vi "PH_ImageOperator.allocate or free img space.vi"(0 "i ref in":refnum<vi>, 2 "Allocate?":bool, 5 "error in (no error)":errorcluster) -> (14 "i ref out":refnum<vi>, 19 "error out":errorcluster)   [LabVIEW 2014, in "PH_ImageOperator.lvlib"]
doc: "This VI is forseen to be used in constructor or destructor. If Allocate? = true is chosen, memory space for several images is allocated. If false is chosen, it is freed."
uses:
  PH_ImageOperator.lvlib
  CS_Core/CSSystem/CSSystemLib/CSSystemLib.lvlib
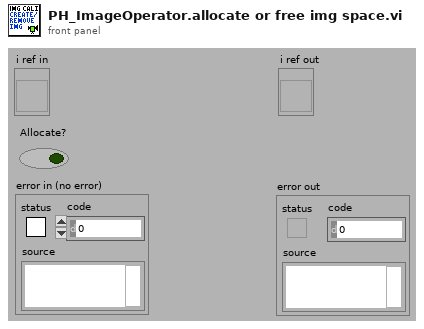
[diagram p1: front panel]
types:
  T1 = typedef "PH_ImageOperator.lvlib/PH_ImageOperator.i attribute.ctl" = cluster{"GUI Refs":cluster{"Delete":refnum<vi>, "Calibration status":refnum<vi>, "BI subtracted":refnum<vi>, "calc Energy":refnum<vi>, "Energy: expected value":refnum<vi>, "Energy: Tolerance":refnum<vi>, "Energy calculated":refnum<vi>, "Energy":refnum<vi>, "calc Beam Anal":refnum<vi>, "Maj Diam 1/esquare":refnum<vi>, "Min Diam 1/esquare":refnum<vi>, "Azi Angle":refnum<vi>, "Min/Maj Diam esquare":refnum<vi>, "Beam analysed":refnum<vi>, "CoG - x":refnum<vi>, "CoG - y":refnum<vi>, "BA: Method":refnum<vi>, "BA: Steps":refnum<vi>, "BA: Factor":refnum<vi>, "calc Traces":refnum<vi>, "Traces: Fit Gauss":refnum<vi>, "Traces calculated":refnum<vi>, "Maj FWHM":refnum<vi>, "Min FWHM":refnum<vi>, "Major Trace":refnum<vi>, "Minor Trace":refnum<vi>, "Maj Fit Order":refnum<vi>, "Min Fit Order":refnum<vi>, "Position calculated":refnum<vi>, "Position":refnum<vi>, "Type":refnum<vi>, "Center":refnum<vi>, "exp - X":refnum<vi>, "exp - Y":refnum<vi>, "Tolerance":refnum<vi>, "f":refnum<vi>, "M":refnum<vi>, "D":refnum<vi>, "q":refnum<vi>, "Dummy Method":refnum<vi>, "Dummy Type":refnum<vi>, "Global On":refnum<vi>, "Traces: No offset":refnum<vi>, "Maj 99%":refnum<vi>, "Min 99%":refnum<vi>, "GUI FF Image":refnum<vi>, "calc Fill Factor":refnum<vi>, "FF calculated":refnum<vi>, "Fill Factor: Filter?":refnum<vi>, "FF: Damage Threshold":refnum<vi>, "FF: Threshold":refnum<vi>, "FF: max allow. Energy":refnum<vi>, "FF: Fillfactor":refnum<vi>, "Calibration data":refnum<vi>}, "List of GUIs":string[], "Calibration":cluster{"Status":T2, "Calibration data":T3, "Calibration Data File":path}, "Final Image":cluster{"BI Subtraction Failure":bool}, "Energy":cluster{"on":bool, "expected value [mJ]":dbl, "Tolerance [%]":dbl, "State":T2, "Energy [mJ]":dbl, "Unit":string, "calculated @":timestamp}, "Beam Analysis":cluster{"on":bool, "Data":T4, "Method":bool, "Steps":i32, "Factor":i32, "ROI":cluster{"Left":i32, "Top":i32, "Right":i32, "Bottom":i32}, "analysed @":timestamp}, "Trace Analysis":cluster{"on":bool, "Fit on":bool, "Maj FWHM":dbl, "Min FWHM":dbl, "Maj Fit Order":i32, "Min Fit Order":i32, "No Offset":bool, "Maj 99%":dbl, "Min 99%":dbl, "Traces":cluster{"XScaleName":string, "Y Scale Minimum":sgl, "Y Scale Maximum":sgl, "X Scale Minimum":sgl, "X Scale Maximum":sgl, "Traces":cluster{"Index":sgl[], "Trace":dbl[]}[]}[], "analysed @":timestamp}, "Position Analysis":cluster{"on":bool, "exp - X":i32, "exp - Y":i32, "focal length [mm]":dbl, "Magnification":dbl, "Delta":dbl, "Theta":dbl, "Tolerance":dbl, "Type":bool, "analysed @":timestamp}, "Fill Factor":cluster{"on":bool, "Filter on?":bool, "Threshold":dbl, "Damage Threshold [J/cm²]":dbl, "Fillfactor":dbl, "Max. allowed Energy [J]":dbl, "calculated @":timestamp}, "Statistician Service ID":i32, "Images":cluster{"Background":T5, "OP":T5, "GUI":T5, "BA: ROI":T5, "Trace: Turn":T5, "FF: Main":T5, "FF: Help":T5, "PSDB: BG":T5, "PSDB: OP":T5, "PSDB: FF":T5}}
  T2 = typedef "PH_StatusHandler.lvlib/PH_StatusHandler.Status.ctl" = i16
  T3 = typedef "PH_ImageCalibrator.lvlib/PH_ImageCalibrator.Calibration Data.ctl" = cluster{"Date":string, "Time":string, "Cam Settings":cluster{"Cam ID":string, "Gain":dbl, "Brightness":dbl, "Shutter":dbl, "Cam Error":bool, "Mode":i32}, "Background Image":cluster{"Image":dbl[][], "Image Error":bool}, "Linear Calibration":cluster{"Calibration Factor":dbl, "not mm or mrad":bool}, "Energy Calibration":cluster{"Calibration Factor":dbl, "no mJ":bool}}
  T4 = typedef "PH_ImageOperator.lvlib/PH_ImageOperator.Beam Analysis Data.ctl" = cluster{"CoG-x":sgl, "CoG-y":sgl, "Maj Dim":dbl, "Min Dim":dbl, "Ellipticity":dbl, "Azimuth Angle [rad]":dbl, "Azi Angle rel to Maj?":bool}
  T5 = typedef "IMAQ Image.ctl" = refnum<image>
  T6 = cluster{"Background":T5, "OP":T5, "GUI":T5, "BA: ROI":T5, "Trace: Turn":T5, "FF: Main":T5, "FF: Help":T5, "PSDB: BG":T5, "PSDB: OP":T5, "PSDB: FF":T5}
  T7 = typedef "Image Type" = u32
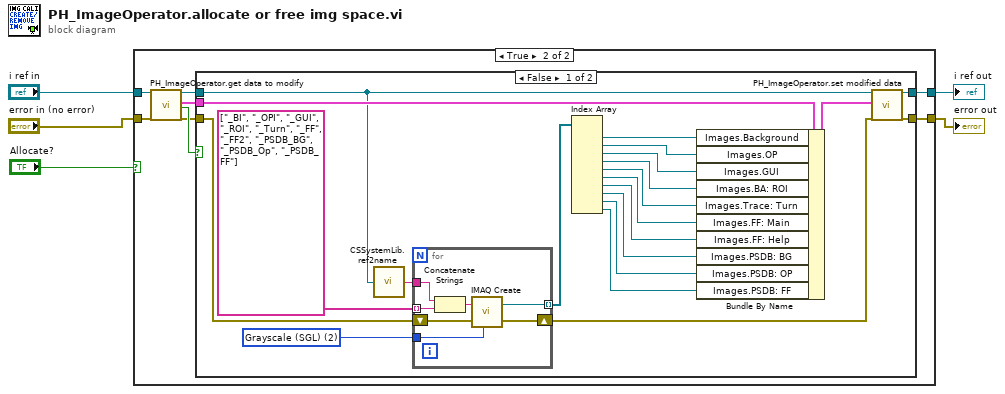
[diagram p0: block diagram]
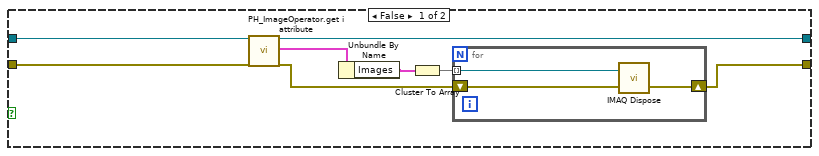
[diagram p2: hidden frame]
diagram:
  n1 = case shown="True" "Allocate?" {
    tunnel: [w8 w23] -> w5
    tunnel: [w10 w22] -> w4
    tunnel: "error in (no error)" -> [w13 w19]
    tunnel: "i ref in" -> [w12 w18]
    frame False {
      n2 = call "PH_ImageOperator.get i attribute.vi"("i ref in"=w12, "error in (no error)"=w13) -> ("i ref out"=w10:refnum<vi>, "i attribute"=w11:T1, "error out"=w9:errorcluster)  [unwired: 15 in]
      n3 = Unbundle By Name(w11) -> ("Images"=w7:T6)
      n4 = Cluster To Array(cluster=w7) -> (array=w6:T5[])
      n5 = for {
        shift-right: [w15] -> w8
        shift-left: w9 -> [w16]
        tunnel: w6 -> [w14] mode=indexing
        n6 = call "IMAQ Dispose"("Image"=w14, "error in (no error)"=w16) -> ("error out"=w15:errorcluster)  [unwired: 4 in]
      }
    }
    frame True {
      n7 = call "PH_ImageOperator.get data to modify.vi"("i ref in"=w18, "error in (no error)"=w19) -> ("i ref out"=w21:refnum<vi>, "i attribute"=w17:T1, "timed out"=w24:bool, "error out"=w20:errorcluster)  [unwired: 14 in]
      n8 = case shown="False" w24 {
        tunnel: w20 -> [w40 w53]
        tunnel: w21 -> [w32 w54]
        tunnel: [w45 w54] -> w22
        tunnel: [w44 w53] -> w23
        tunnel: w17 -> [w43 _]
        frame False {
          w35 = T7 2 items=["Grayscale (U8)", "Grayscale (I16)", "Grayscale (SGL)", "Complex (CSG)", "RGB (U32)", "HSL (U32)", "RGB (U64)"] ("Image Type")
          n9 = call "CSSystemLib.ref2name.vi"("obj refnum"=w32) -> ("name"=w31:string)
          n10 = for {
            shift-right: [w52] -> w41
            shift-left: w40 -> [w51]
            tunnel: [w46] -> w39 mode=indexing
            tunnel: string[] ["_BI", "_OPI", "_GUI", "_ROI", "_Turn", "_FF", "_FF2", "_PSDB_BG", "_PSDB_Op", "_PSDB_FF"] -> [w48] mode=indexing
            tunnel: w35 -> [w50]
            tunnel: w31 -> [w49]
            n11 = Concatenate Strings(w49, w48) -> (w47:string)
            n12 = call "IMAQ Create"("Image Name"=w47, "Image Type"=w50, "error in (no error)"=w51) -> ("New Image"=w46:T5, "error out"=w52:errorcluster)  [unwired: 2 in]
          }
          n13 = Index Array(array=w39) -> (element #1=w37:T5, element #2=w36:T5, element #3=w34:T5, element #4=w33:T5, element #5=w30:T5, element #6=w29:T5, element #7=w28:T5, element #8=w27:T5, element #9=w26:T5, element #10=w25:T5)  [unwired: 10 in]
          n14 = Bundle By Name(cluster=w43, "Images.Background"=w37, "Images.OP"=w36, "Images.GUI"=w34, "Images.BA: ROI"=w33, "Images.Trace: Turn"=w30, "Images.FF: Main"=w29, "Images.FF: Help"=w28, "Images.PSDB: BG"=w27, "Images.PSDB: OP"=w26, "Images.PSDB: FF"=w25) -> (w42:T1)
          n15 = call "PH_ImageOperator.set modified data.vi"("i ref in"=w32, "i attribute"=w42, "error in (no error)"=w41) -> ("i ref out"=w45:refnum<vi>, "error out"=w44:errorcluster)  [unwired: 15 in]
        }
        frame True {
        }
      }
    }
  }
  "error out" <- w5
  "i ref out" <- w4
